vi "Set ServerEvent.vi"(7 "Complete Call (T)":bool=TRUE, 8 "error in (no error)":errorcluster, 10 "ServerEvent_Data":T2, 11 "gRPCid in":T1) -> (0 "error out":errorcluster)   [LabVIEW 2019]
uses:
  ServerEvent_Data.ctl
  gRPC interface/Server API/typeDefs/grpcId.ctl
  7bdd4605-c7f7-42bf-87d0-91e104daf0dd.vi
  <vilib>/Utility/error.llb/Error Cluster From Error Code.vi
  gRPC interface/gprc-lvsupport.lvlib
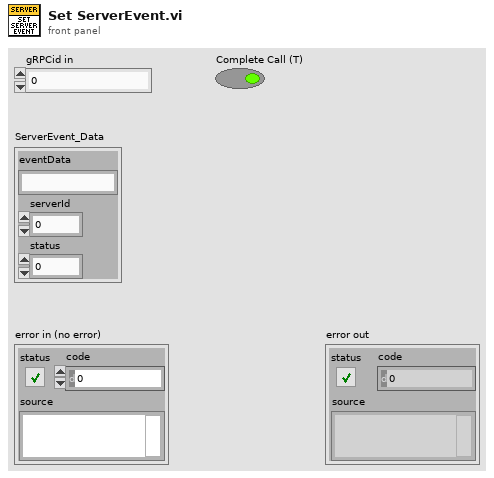
[diagram p1: front panel]
types:
  T1 = typedef "gprc-lvsupport.lvlib/grpcId.ctl" = u64
  T2 = typedef "ServerEvent_Data.ctl" = cluster{"eventData":string, "serverId":i32, "status":i32}
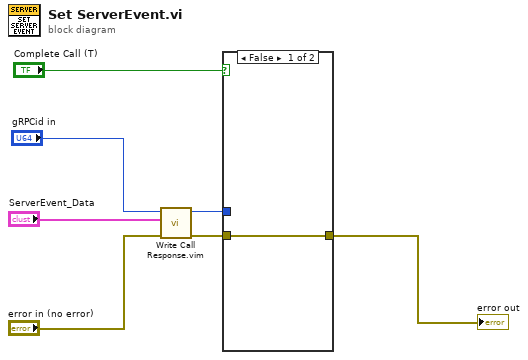
[diagram p0: block diagram]
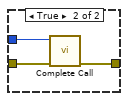
[diagram p2: hidden frame]
diagram:
  n1 = call "Write Call Response.vim"("error in (no error)"="error in (no error)", "Response Data"="ServerEvent_Data", "gRPCid in"="gRPCid in") -> ("error out"=w3:errorcluster, "gRPCid"=w4:T1)  [unwired: 7 in]
  n2 = case shown="False" "Complete Call (T)" {
    tunnel: [w8 w11] -> w1
    tunnel: w3 -> [w8 w10]
    tunnel: w4 -> [_ w9]
    frame False {
    }
    frame True {
      n3 = call "Complete Call.vi"("gRPCid"=w9, "error in (no error)"=w10) -> ("error out"=w11:errorcluster)  [unwired: 8 in]
    }
  }
  "error out" <- w1
